vi "FABR-Initialize.vi"(0 "Params":T4={"Stimulus"={"Ear"=enum."Left", "Start (kHz)"=0.0, "Stop (kHz)"=16.0, "Step (oct)"=5.0, "Start (dB)"=0, "Stop (dB)"=30, "Step (dB)"=5, "Rep rate (/sec)"=30.0, "Alternate Polarity"=FALSE, "Skip (oct)"=0.0}, "Response"={"Gain"=1.0, "Averages"=0, "Window (ms)"=0.0}, "Hidden"={"AI Samp Rate Hz"=10000.0, "AO Samp Rate Hz"=512.0, "Duration (ms)"=8.5, "Ramp (ms)"=8.5, "Frame size (s)"=0.0}, "Reject"=0.0} {"Response"."Window (ms)" format="%.2f"; "Stimulus"."Start (kHz)" step=5.0; "Stimulus"."Start (dB)" step=5}, 1 "State":T9) -> (4 "Runtime":T8, 6 "Tickets out":T1[](array[typedef]), 8 "SCL":T2[](array[typedef]), 13 "Analysis":T3, 15 "error out":errorcluster)   [LabVIEW 2020]
uses:
  CFTS Main Panel SubVIs/CFTS-Experiment State.ctl
  Typedefs/FABR-Runtime Data.ctl
  Typedefs/FABR-Parameters.ctl
  Typedefs/FABR-Stimulus.ctl
  Typedefs/FABR-Response.ctl
  Typedefs/FABR-Hidden Params.ctl
  Typedefs/FABR-Analysis State.ctl
  Typedefs/FABR-Stimulus Condition.ctl
  Typedefs/FABR-Stimulus Ticket.ctl
panel:
  in  "error in (no error)":errorcluster
  # "Freq X Level X Time"
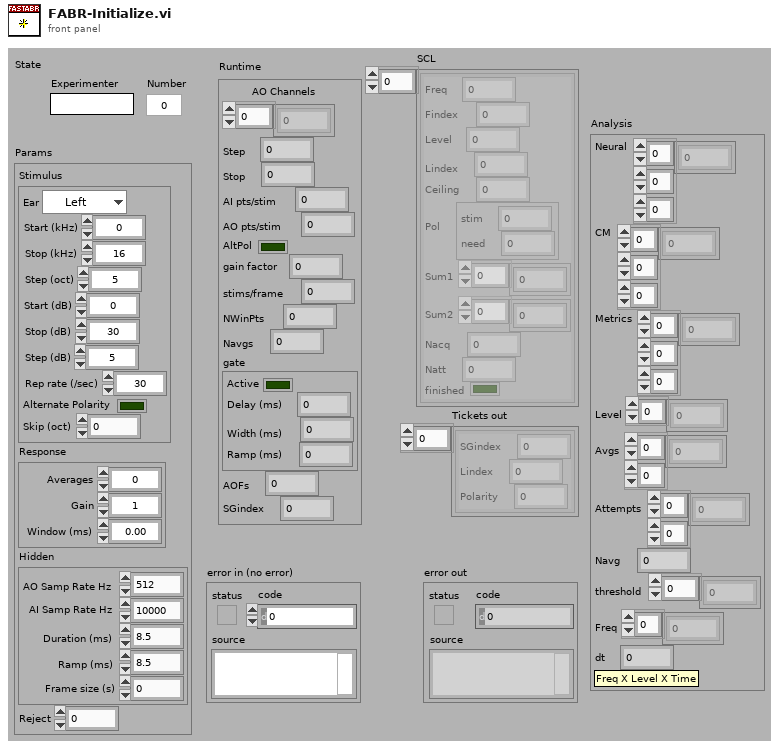
[diagram p1: front panel]
types:
  T1 = typedef "FABR-Stimulus Ticket.ctl" = cluster{"SGindex":i32, "Lindex":i32, "Polarity":i32}
  T2 = typedef "FABR-Stimulus Condition.ctl" = cluster{"Freq":dbl, "Findex":i32, "Level":dbl, "Lindex":i32, "Ceiling":dbl, "Pol":cluster{"stim":i32, "need":i32}, "Sum1":dbl[], "Sum2":dbl[], "Nacq":i32, "Natt":i32, "finished":bool}
  T3 = typedef "FABR-Analysis State.ctl" = cluster{"Neural":dbl[][][], "CM":dbl[][][], "Metrics":dbl[][][], "Level":dbl[], "Avgs":i32[][], "Attempts":i32[][], "Navg":i32, "threshold":dbl[], "Freq":dbl[], "dt":dbl}
  T4 = typedef "FABR-Parameters.ctl" = cluster{"Stimulus":T5, "Response":T6, "Hidden":T7, "Reject":dbl}
  T5 = typedef "FABR-Stimulus.ctl" = cluster{"Ear":enum16{"Right", "Left"}, "Start (kHz)":dbl, "Stop (kHz)":dbl, "Step (oct)":dbl, "Start (dB)":i32, "Stop (dB)":i32, "Step (dB)":i32, "Rep rate (/sec)":dbl, "Alternate Polarity":bool, "Skip (oct)":dbl}
  T6 = typedef "FABR-Response.ctl" = cluster{"Gain":dbl, "Averages":i32, "Window (ms)":sgl}
  T7 = typedef "FABR-Hidden Params.ctl" = cluster{"AI Samp Rate Hz":dbl, "AO Samp Rate Hz":dbl, "Duration (ms)":dbl, "Ramp (ms)":dbl, "Frame size (s)":dbl}
  T8 = typedef "FABR-Runtime Data.ctl" = cluster{"AO Channels":i32[], "Step":dbl, "Stop":i32, "AI pts/stim":i32, "AO pts/stim":i32, "AltPol":bool, "gain factor":dbl, "stims/frame":i32, "NWinPts":i32, "Navgs":i32, "gate":cluster{"Active":bool, "Delay (ms)":dbl, "Width (ms)":dbl, "Ramp (ms)":dbl}, "AOFs":dbl, "SGindex":i32}
  T9 = typedef "CFTS-Experiment State.ctl" = cluster{"Experimenter":string, "Number":u32, "Right":string, "Left":string, "Data Folder":path, "State File":path, "Version Info":string, "End Exposure Time":dbl, "Exposure Duration":string, "Run #":cluster{"CAP":i16, "ABR":i16, "DP":i16, "VsEP":i16, "MeasSeq":i16, "SubSeq":i16, "SFOAE":i16}}
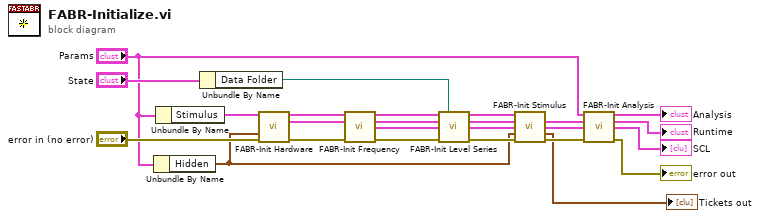
[diagram p0: block diagram]
diagram:
  n1 = Unbundle By Name("Params") -> ("Hidden"=w10:T7)
  n2 = Unbundle By Name("Params") -> ("Stimulus"=w22:T5)
  n3 = Unbundle By Name("State") -> ("Data Folder"=w24:path)
  n4 = call "FABR-Init Hardware.vi"("Stimulus"=w22, "Hidden"=w10, "error in (no error)"="error in (no error)") -> ("Stimulus thru"=w21:T5, "Runtime"=w20:T8, "error out"=w16:errorcluster)  [unwired: 9 in, 1 out]
  n5 = call "FABR-Init Frequency.vi"("Stimulus"=w21, "Runtime in"=w20, "error in (no error)"=w16) -> ("Stimulus thru"=w19:T5, "Runtime out"=w18:T8, "SCL"=w17:T2[], "error out"=w15:errorcluster)  [unwired: 9 in]
  n6 = call "FABR-Init Level Series.vi"("Stimulus"=w19, "Data Folder"=w24, "Runtime In"=w18, "SCL in"=w17, "error in (no error)"=w15) -> ("Stimulus thru"=w14:T5, "Runtime Out"=w12:T8, "SCL out"=w11:T2[], "error out"=w13:errorcluster)  [unwired: 7 in]
  n7 = call "FABR-Init Stimulus.vi"("Stimulus"=w14, "Runtime In"=w12, "SCL"=w11, "Hidden"=w10, "error in (no error)"=w13) -> ("Runtime Out"=w8:T8, "SCL thru"=w3:T2[], "Tickets out"=→"Tickets out":T1[], "error out"=w7:errorcluster)  [unwired: 7 in]
  n8 = call "FABR-Init Analysis.vi"("Params"="Params", "Runtime in"=w8, "SCL in"=w3, "error in (no error)"=w7) -> ("Analysis"=→"Analysis":T3, "Runtime out"=→"Runtime":T8, "SCL out"=→"SCL":T2[], "error out"=→"error out":errorcluster)  [unwired: 8 in]
